vi "Compute_OD.vi"(0 "dark":u16[][](array[numeric]), 1 "flat":u16[][](array[numeric]), 2 "atoms":u16[][](array[numeric]), 3 "ctx in":T1 format="%.0x", 4 "params":T2, 5 "identity":string="bias", 6 "timeout":u32=30000) -> (7 "error out":errorcluster, 8 "alpha":dbl, 9 "N":dbl, 10 "OD":sgl[][](array[numeric]))   [LabVIEW 2010]
uses:
  <vilib>/addons/zeromq/pointer.ctl
panel:
  in  "error in":errorcluster
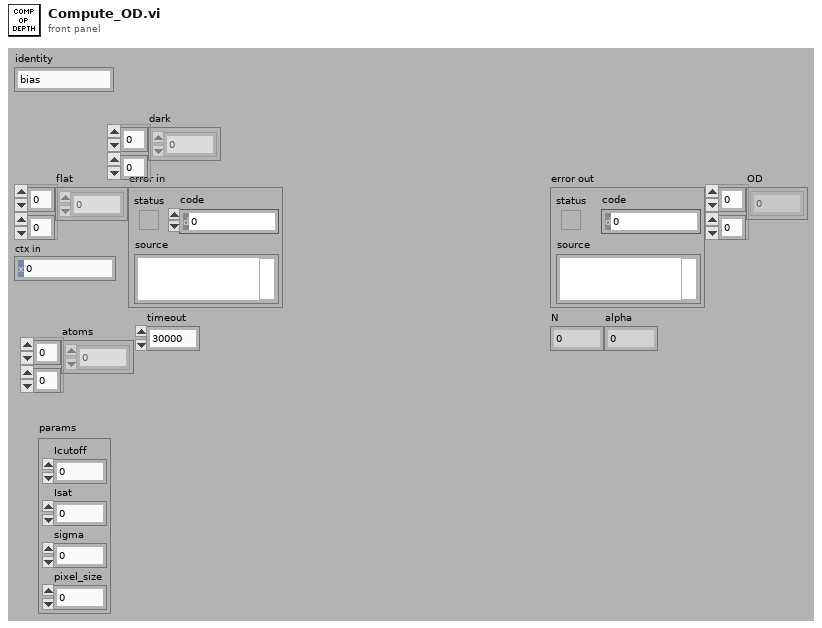
[diagram p1: front panel]
types:
  T1 = typedef "pointer.ctl" = u64
  T2 = cluster{"Icutoff":dbl, "Isat":dbl, "sigma":dbl, "pixel_size":dbl}
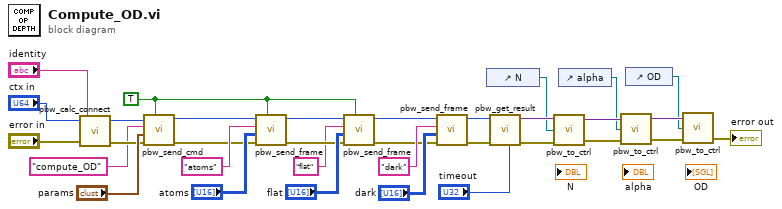
[diagram p0: block diagram]
diagram:
  w5 = TRUE ("more? (F)")
  n1 = call <userlib>:"pbw_calc_connect.vi"("error in"="error in", "identity"="identity", "ctx in"="ctx in") -> ("error out"=w8:errorcluster, "socket out"=w7:T1)  [unwired: 1 in]
  n2 = call <vilib>:"pbw_send_cmd.vi"("more? (F)"=w5, "error in"=w8, "cluster"="params", "command"="compute_OD" ("data"), "socket in"=w7) -> ("error out"=w11:errorcluster, "socket out"=w12:u64)  [unwired: 2 in]
  n3 = call <vilib>:"pbw_send_frame.vi"("more? (F)"=w5, "error in"=w11, "data"="atoms", "name"="atoms", "socket in"=w12) -> ("error out"=w30:errorcluster, "socket out"=w31:u64)  [unwired: 2 in]
  n4 = call <vilib>:"pbw_send_frame.vi"("more? (F)"=w5, "error in"=w30, "data"="flat", "name"="flat", "socket in"=w31) -> ("error out"=w23:errorcluster, "socket out"=w24:u64)  [unwired: 2 in]
  n5 = call <vilib>:"pbw_send_frame.vi"("error in"=w23, "data"="dark", "name"="dark", "socket in"=w24) -> ("error out"=w3:errorcluster, "socket out"=w4:u64)  [unwired: 3 in]
  n6 = control-ref of="N"() -> (w16:refnum<vi>)
  n7 = call <vilib>:"pbw_get_result.vi"("error in"=w3, "socket in"=w4, "timeout"="timeout") -> ("error out"=w21:errorcluster, "return vals"=w22:variant)  [unwired: 4 in]
  n8 = call <vilib>:"pbw_to_ctrl.vi"("error in"=w21, "control"=w16, "variant w attribs"=w22) -> ("error out"=w17:errorcluster, "duplicate variant"=w18:variant)  [unwired: 1 out]
  n9 = control-ref of="alpha"() -> (w15:refnum<vi>)
  n10 = call <vilib>:"pbw_to_ctrl.vi"("error in"=w17, "control"=w15, "variant w attribs"=w18) -> ("error out"=w19:errorcluster, "duplicate variant"=w20:variant)  [unwired: 1 out]
  n11 = control-ref of="OD"() -> (w14:refnum<vi>)
  n12 = call <vilib>:"pbw_to_ctrl.vi"("error in"=w19, "control"=w14, "variant w attribs"=w20) -> ("error out"=→"error out":errorcluster)  [unwired: 2 out]
